vi "Initialize.vi"(8 "error in (no error)":errorcluster, 10 "Configuration":T1, 11 "TCP_Streamer_Subscriber in":refnum<class "TCP_Streamer_Subscriber.lvclass">) -> (0 "error out":errorcluster, 3 "TCP_Streamer_Subscriber out":refnum<class "TCP_Streamer_Subscriber.lvclass">)   [LabVIEW 2021, in "TCP_Streamer_Subscriber.lvclass"]
uses:
  TCP_Streamer_Subscriber.lvclass
  TCP_Streamer_Subscriber.lvclass/TCP_Streamer_Subscriber.ctl
  Typedef/State.ctl
  Typedef/Configuration.ctl
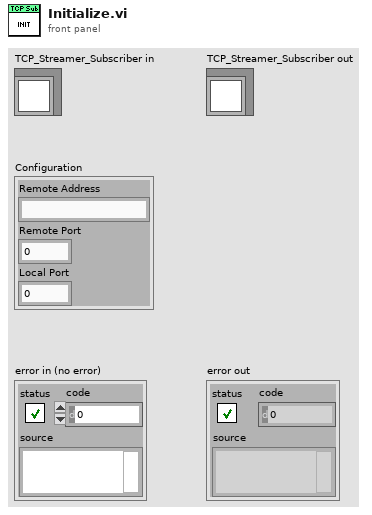
[diagram p1: front panel]
types:
  T1 = typedef "TCP_Streamer_Subscriber.lvclass/Configuration.ctl" = cluster{"Remote Address":string, "Remote Port":u16, "Local Port":u16}
  T2 = typedef "TCP_Streamer_Subscriber.lvclass/State.ctl" = enum16{"Stopped", "Connecting", "Receiving"}
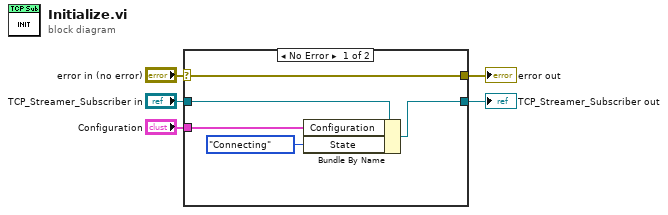
[diagram p0: block diagram]
diagram:
  n1 = case shown="No Error" "error in (no error)" {
    selector: "error in (no error)" -> [w10 w12]
    tunnel: [w10 w12] -> w4
    tunnel: [w8 w11] -> w2
    tunnel: "TCP_Streamer_Subscriber in" -> [w9 w11]
    tunnel: "Configuration" -> [w7 _]
    frame No Error {
      n2 = Bundle By Name(cluster=w9, "Configuration"=w7, "State"=State."Connecting") -> (w8:refnum<class "TCP_Streamer_Subscriber.lvclass">)
    }
    frame Error {
    }
  }
  "error out" <- w4
  "TCP_Streamer_Subscriber out" <- w2
